vi "报警判断 (子VI).vi"(11 "后左滚筒右轴承":dbl) -> (3 "布尔":bool)   [LabVIEW 2016]
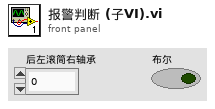
[diagram p1: front panel]
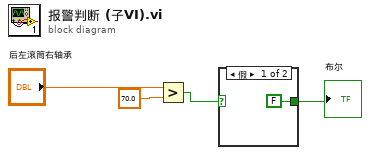
[diagram p0: block diagram]
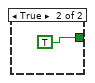
[diagram p2: hidden frame]
diagram:
  n1 = Greater?(x="后左滚筒右轴承", y=70.0) -> (0:w3:bool)
  n2 = case shown="假" w3 {
    tunnel: [FALSE TRUE] -> w4
    frame False {
    }
    frame True {
    }
  }
  "布尔" <- w4
